vi "MeasurementItems_GetChannels.vi"(8 "error in (no error)":errorcluster, 11 "OXY_SCPI Reseource In":refnum<visa-resource-name>) -> (0 "error out":errorcluster, 1 "communication_data":T1, 2 "Channel Item List":string[](array[string]), 3 "OXY_SCPI Reseource Out":refnum<visa-resource-name>)   [LabVIEW 2018, in "OXYGEN.lvlib"]
doc: "Query numeric data output items."
uses:
  OXYGEN.lvlib
  TypeDefs/Cluster_RawCommData.ctl
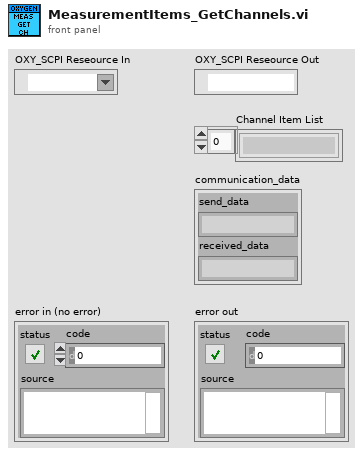
[diagram p1: front panel]
types:
  T1 = typedef "OXYGEN.lvlib/Cluster_RawCommData.ctl" = cluster{"send_data":string, "received_data":string}
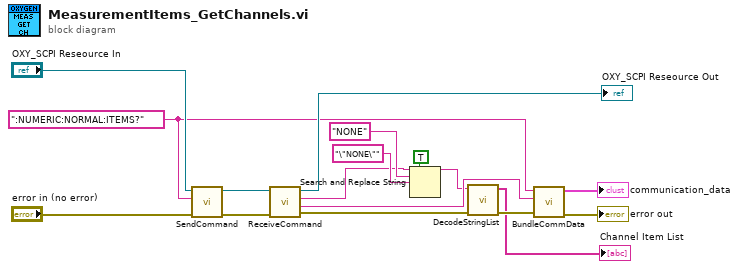
[diagram p0: block diagram]
diagram:
  w7 = ":NUMERIC:NORMAL:ITEMS?" ("String to Send")
  n1 = call "SendCommand.vi"("error in (no error)"="error in (no error)", "String to Send"=w7, "OXY_SCPI Reseource In"="OXY_SCPI Reseource In") -> ("error out"=w17:errorcluster, "OXY_SCPI Reseource Out"=w16:refnum<visa-resource-name>)  [unwired: 7 in]
  n2 = call "ReceiveCommand.vi"("error in (no error)"=w17, "OXY_SCPI Reseource In"=w16) -> ("error out"=w10:errorcluster, "received Data with Header"=w4:string, "received Data"=w2:string, "OXY_SCPI Reseource Out"=→"OXY_SCPI Reseource Out":refnum<visa-resource-name>)  [unwired: 6 in]
  n3 = Search and Replace String(replace all?=TRUE ("replace all? (F)"), input string=w2, search string="NONE", replace string="\"NONE\"" ("replace string (\"\")")) -> (result string=w3:string)  [unwired: 4 in, 3 out]
  n4 = call "DecodeStringList.vi"("error in (no error)"=w10, "String List (\"<STR1>\",\"<STR2>\",...)"=w3) -> ("error out"=w9:errorcluster, "String as Array"=→"Channel Item List":string[])  [unwired: 8 in]
  n5 = call "BundleCommData.vi"("error in (no error)"=w9, "received_data"=w4, "send_data"=w7) -> ("error out"=→"error out":errorcluster, "communication_data"=→"communication_data":T1)  [unwired: 7 in]
